vi "等待-读写间隔.vi"(6 "轮询间隔（10ms）":u32=10, 7 "确定次数（1）":u32=1, 8 "error in":errorcluster={"status"=TRUE, "code"=0, "source"=""}, 9 "设置超时(默认-1,单位ms)":i32=-1, 10 "等待字节数(4096)":u32=4096, 11 "VISA资源名i":refnum<visa-resource-name>) -> (0 "error out":errorcluster, 1 "等待时间ms":u32, 2 "读取字节数":u32=17, 3 "VISA资源名o":refnum<visa-resource-name>, 4 "超时？":bool)   [LabVIEW 2017]
panel:
  in  "读取结束？":bool
  out ">=字节数？":bool
  in  "标志-超时？":bool
  in  "停止按钮":bool
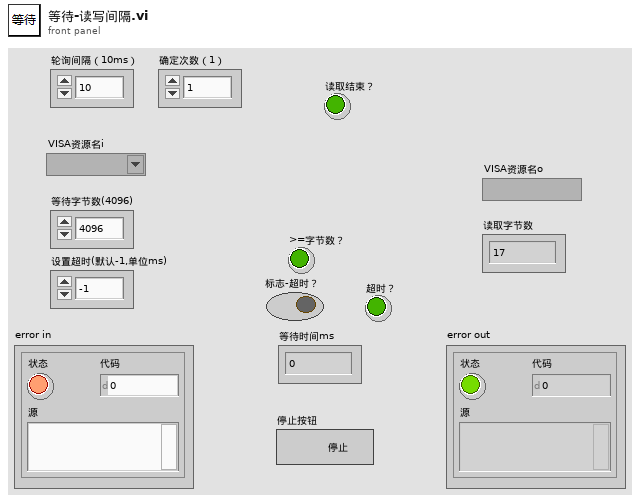
[diagram p1: front panel]
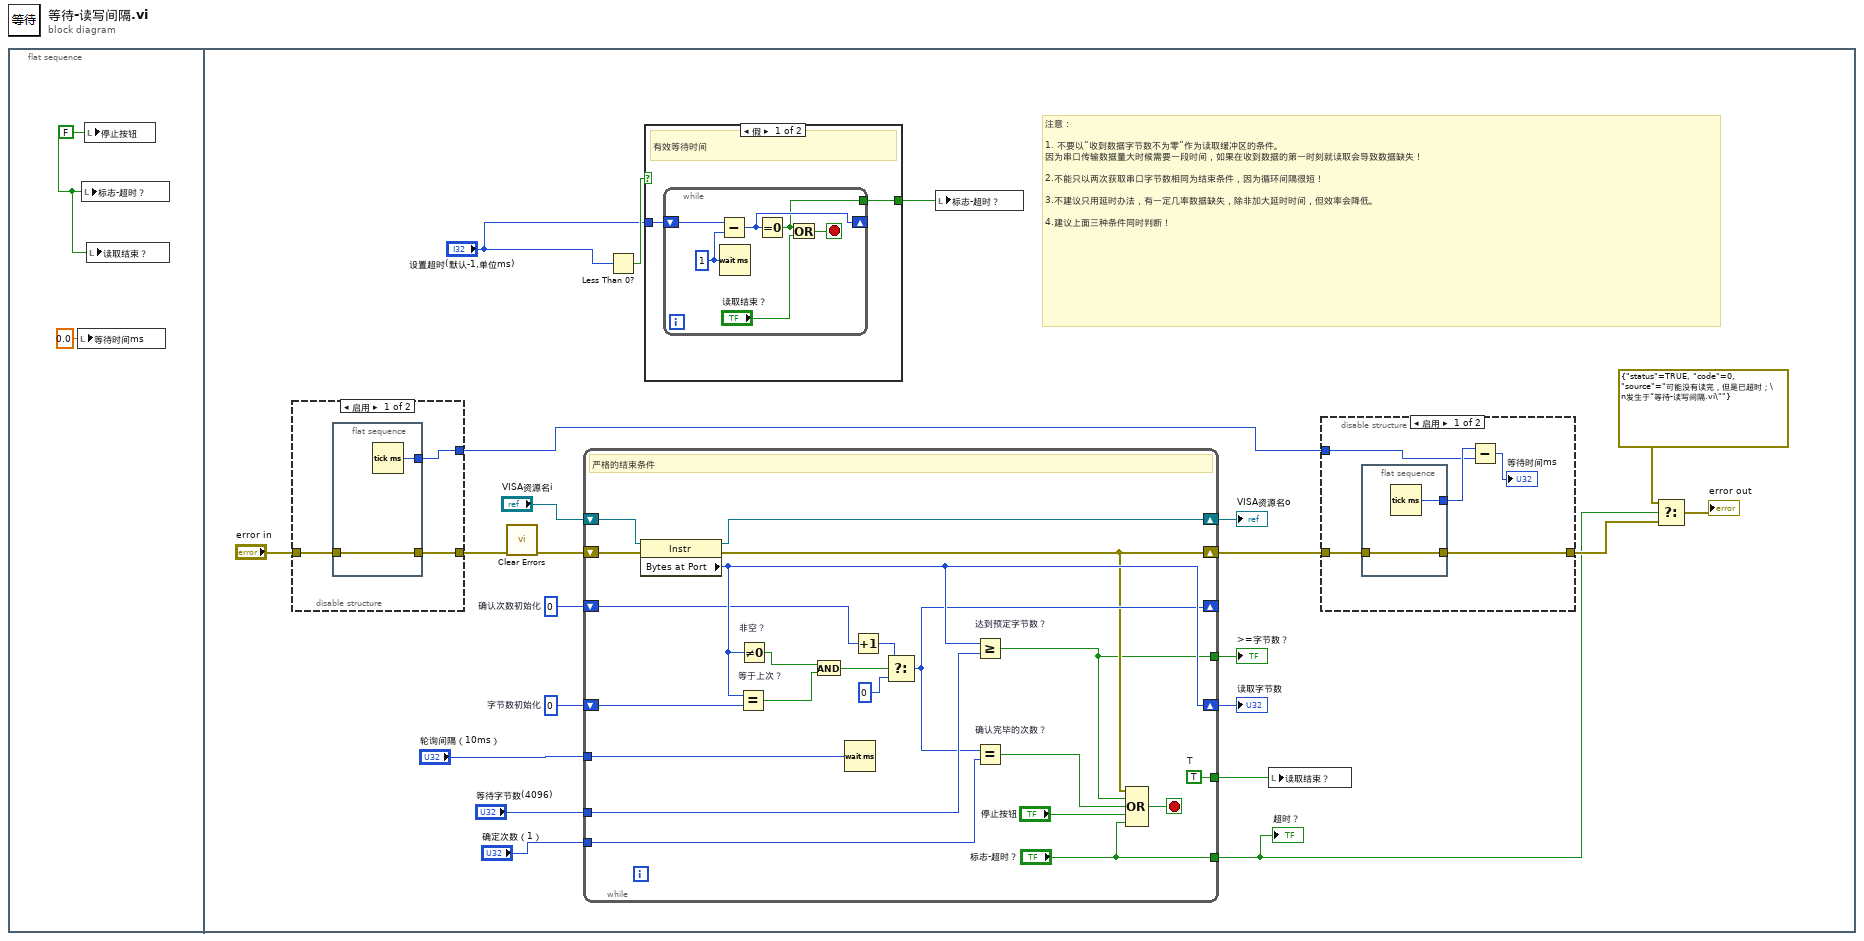
[diagram p0: block diagram]
diagram:
  n1 = flat-sequence {
    frame #0 {
      w1 = FALSE ("停止按钮")
      n2 = local write "等待时间ms"(0.0 ("读取时间s")) -> ()
      n3 = local write "标志-超时？"(w1) -> ()
      n4 = local write "停止按钮"(w1) -> ()
      n5 = local write "读取结束？"(w1) -> ()
    }
    frame #1 {
      w17 = u32 0  # 确认次数初始化
      w20 = u32 0  # 字节数初始化
      # "注意：\n\n1. 不要以“收到数据字节数不为零”作为读取缓冲区的条件。\n因为串口传输数据量大时候需要一段时间，如果在收到数据的第一时刻就读取会导致数据缺失！\n\n2.不能只以两次获取串口字节数相同为结束条件，因为循环间隔很短！\n\n3.不建议只用延时办法，有一定几率数据缺失，除非加大延时时间，但效率会降低。\n\n4.建议上面三种条件同时判断！"
      n6 = disable-structure shown="启用" {
        disable-tunnel: [w43 w46] -> w15
        disable-tunnel: [w42 _] -> w21
        disable-tunnel: "error in" -> [w41 w46]
        frame Enabled {
          n7 = flat-sequence {
            tunnel: [w45] -> w43
            tunnel: w41 -> [w45]
            tunnel: [w44] -> w42
            frame #0 {
              n8 = Tick Count (ms)() -> (millisecond timer value=w44:u32)
            }
          }
        }
        frame Disabled {
        }
      }
      n9 = call <vilib>:"Clear Errors.vi"("error in (no error)"=w15) -> ("error out"=w5:errorcluster)  [unwired: 5 in, 1 out]
      n10 = while {
        shift-right: [w68] -> w19
        shift-left: "VISA资源名i" -> [w66]
        tunnel: "等待字节数(4096)" -> [w64]
        shift-right: [w54] -> w14
        shift-left: w5 -> [w65]
        shift-right: [w62] -> w18
        shift-left: w20 -> [w61]
        shift-right: [w59] -> _
        shift-left: w17 -> [w58]
        tunnel: [w53] -> w16
        tunnel: ["标志-超时？"] -> w3
        tunnel: [w49] -> w8
        tunnel: "轮询间隔（10ms）" -> [w48]
        tunnel: "确定次数（1）" -> [w47]
        stop <- w50 stop-if-true
        w49 = TRUE  # T
        # "严格的结束条件"
        n11 = property class="Instr"(reference=w66, error in=w65) -> (reference out=w68:refnum<visa-resource-name>, error out=w54:errorcluster, "Bytes at Port"=w62:u32)
        n12 = Equal? "等于上次？"(x=w62, y=w61) -> (x = y?=w57:bool)
        n13 = Not Equal To 0? "非空？"(x=w62) -> (x != 0?=w63:bool)
        n14 = And(x=w63, y=w57) -> (x .and. y?=w56:bool)
        n15 = Wait (ms)(milliseconds to wait=w48) -> ()  [unwired: 1 out]
        n16 = Increment(x=w58) -> (x+1=w60:u32)
        n17 = Select(t=w60, s=w56, f=u32 0) -> (s? t:f=w59:u32)
        n18 = Greater Or Equal? "达到预定字节数？"(x=w62, y=w64) -> (x >= y?=w53:bool)
        n19 = Equal? "确认完毕的次数？"(x=w59, y=w47) -> (x = y?=w52:bool)
        n20 = Compound Arithmetic op=OR(w54, w53, w52, "停止按钮", "标志-超时？") -> (w50:bool)
      }
      "读取字节数" <- w18
      "VISA资源名o" <- w19
      ">=字节数？" <- w16
      "超时？" <- w3
      n21 = Less Than 0?(x="设置超时(默认-1,单位ms)") -> (x < 0?=w10:bool)
      n22 = case shown="假" w10 {
        tunnel: "设置超时(默认-1,单位ms)" -> [w26 _]
        tunnel: [w25 _] -> w4
        frame False {
          # "有效等待时间"
          n23 = while {
            shift-right: [w29] -> _
            shift-left: w26 -> [w32]
            tunnel: [w27] -> w25
            stop <- w28 stop-if-true
            w31 = 1 ("y")
            n24 = Subtract(x=w32, y=w31) -> (x-y=w29:i32)
            n25 = Wait (ms)(milliseconds to wait=w31) -> ()  [unwired: 1 out]
            n26 = Equal To 0?(x=w29) -> (x = 0?=w27:bool)
            n27 = Or(x=w27, y="读取结束？") -> (x .or. y?=w28:bool)
          }
        }
        frame True {
          # "永不超时"
        }
      }
      n28 = local write "标志-超时？"(w4) -> ()
      n29 = local write "读取结束？"(w8) -> ()
      n30 = disable-structure shown="启用" {
        disable-tunnel: w14 -> [w37 w40]
        disable-tunnel: w21 -> [w35 _]
        disable-tunnel: [w34 w40] -> w13
        frame Enabled {
          n31 = flat-sequence {
            tunnel: w37 -> [w39]
            tunnel: [w39] -> w34
            tunnel: [w38] -> w36
            frame #0 {
              n32 = Tick Count (ms)() -> (millisecond timer value=w38:u32)
            }
          }
          n33 = Subtract(x=w36, y=w35) -> (x-y=→"等待时间ms":u32)
        }
        frame Disabled {
        }
      }
      n34 = Select(t=errorcluster {"status"=TRUE, "code"=0, "source"="可能没有读完，但是已超时；\n发生于“等待-读写间隔.vi\""} ("error in"), s=w3, f=w13) -> (s? t:f=→"error out":errorcluster)
    }
  }
